vi "Save Accelerometer Data.vi"(7 "zero":bool, 8 "error in (no error)":errorcluster, 10 "Accelerometer Data":T1, 11 "tdms file":refnum<k34>) -> (0 "error out":errorcluster, 3 "tdms file out":refnum<k34>)   [LabVIEW 2013]
uses:
  Accelerometer Data.ctl
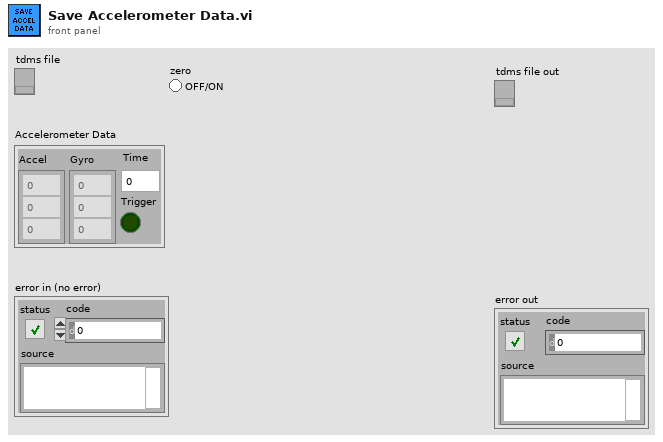
[diagram p1: front panel]
types:
  T1 = typedef "Accelerometer Data.ctl" = cluster{"Accel":dbl[], "Gyro":dbl[], "Time":u64, "Trigger":bool}
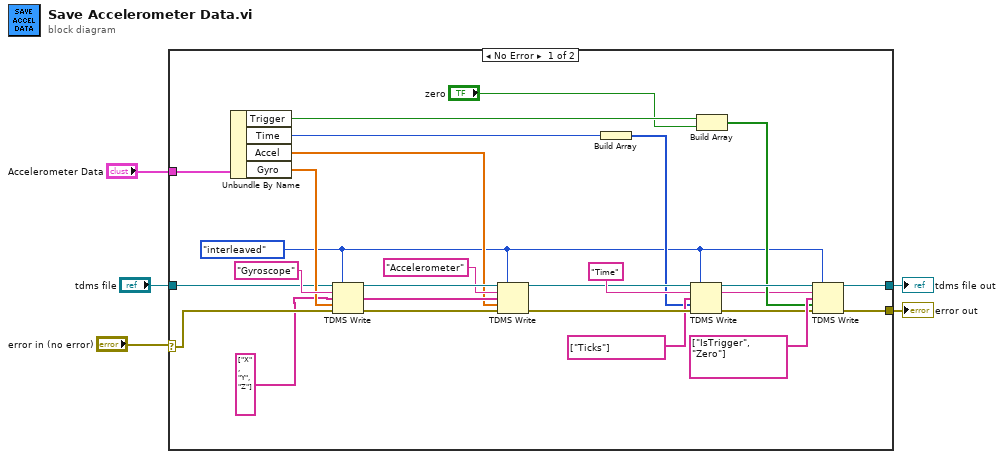
[diagram p0: block diagram]
diagram:
  n1 = case shown="No Error" "error in (no error)" {
    selector: "error in (no error)" -> [w31 w33]
    tunnel: "Accelerometer Data" -> [w30 _]
    tunnel: "tdms file" -> [w26 w34]
    tunnel: [w9 w34] -> w2
    tunnel: [w8 w33] -> w1
    frame No Error {
      w10 = enum16{"decimated", "interleaved"}."interleaved" ("data layout (0:decimated)")
      n2 = Unbundle By Name(w30) -> ("Trigger"=w12:bool, "Time"=w17:u64, "Accel"=w23:dbl[], "Gyro"=w29:dbl[])
      n3 = TDMS Write(0:w26, 1:w10, 5:"Gyroscope" ("group name (Untitled)"), 7:string[] ["X", "Y", "Z"] ("channel name(s)"), 9:w29, 11:w31) -> (4:w28:refnum<k34>, 8:w25:string[], 15:w22:errorcluster)  [unwired: 1 out]
      n4 = TDMS Write(0:w28, 1:w10, 5:"Accelerometer" ("group name (Untitled)"), 7:w25, 9:w23, 11:w22) -> (4:w20:refnum<k34>, 15:w19:errorcluster)  [unwired: 2 out]
      n5 = Build Array(w17) -> (w16:u64[])
      n6 = TDMS Write(0:w20, 1:w10, 5:"Time" ("group name"), 7:string[] ["Ticks"] ("channel name(s)"), 9:w16, 11:w19) -> (4:w14:refnum<k34>, 6:w7:string, 15:w13:errorcluster)  [unwired: 1 out]
      n7 = Build Array(w12, "zero") -> (w11:bool[])
      n8 = TDMS Write(0:w14, 1:w10, 5:w7, 7:string[] ["IsTrigger", "Zero"] ("channel name(s)"), 9:w11, 11:w13) -> (4:w9:refnum<k34>, 15:w8:errorcluster)  [unwired: 2 out]
    }
    frame Error {
    }
  }
  "tdms file out" <- w2
  "error out" <- w1
